vi "Shooting Stars RT Test.vi"() -> ()   [LabVIEW 2021]
uses:
  Display Utilities/Public/Controls/2D Dimensions.ctl
  Neopixel - Host/Public/Controls/RGB Gains.ctl
  Display Utilities/Public/Controls/2D Coordinates.ctl
  Pixel/Pixel.lvclass
  C:/Git/MEMOSFET/myRIO-Neopixel/Source/RT/Display Element/Display Element.lvclass
  <vilib>/numeric/Random Number (Range) U64.vi
  <vilib>/numeric/Random Number (Range) I64.vi
  <vilib>/numeric/sub_Random U32.vi
  <vilib>/FPGAPlugInAG/myRIO-1900/niLvFpga_Open_myRIO-1900.vi
  <vilib>/rvi/interface/common/dynamic/niFpgaDynamicAddResources.vi
  <vilib>/FPGAPlugInAG/Dynamic/niLvFpga_Close_Dynamic.vi
  <vilib>/rvi/interface/nirviOpenFPGA/nirviOpenFPGA.xnode
  FPGA Bitfiles/Test Neopixel.lvbitx
  <vilib>/rvi/interface/nirviCloseFPGA/nirviCloseFPGA.xnode
  Neopixel - Host/Neopixel - Host.lvclass
  Display Utilities/Display Utilities.lvlib
  Display Manager/Display Manager.lvclass
panel:
  out "Frame":u32[][](array[colorbox])
  in  "Intensity":sgl(slide)=0.5 scale=0.0..1.0
  in  "FPS":u32(slide)=40 scale=0.0..500.0
  in  "stop":bool
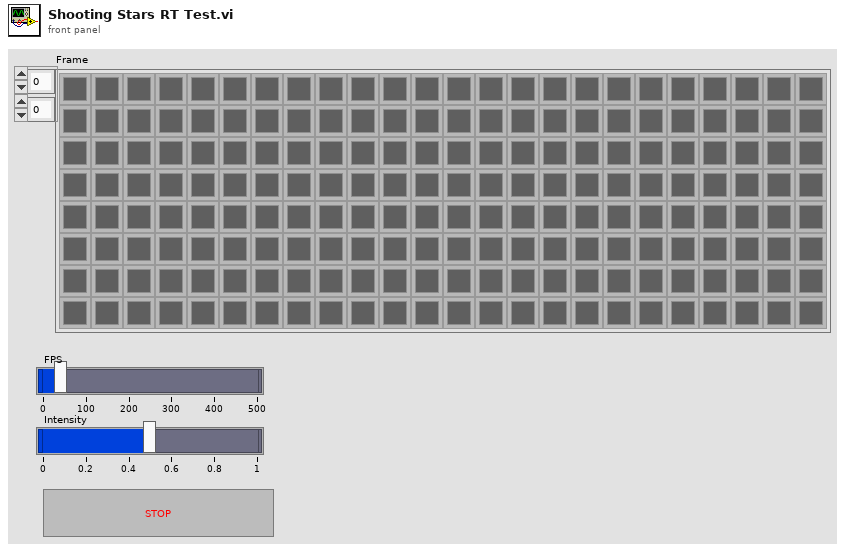
[diagram p1: front panel]
types:
  T1 = typedef "Display Utilities.lvlib/2D Dimensions.ctl" = cluster{"Width":i32, "Height":i32}
  T2 = typedef "Neopixel - Host.lvclass/RGB Gains.ctl" = cluster{"Red":sgl, "Green":sgl, "Blue":sgl}
  T3 = typedef "Display Utilities.lvlib/2D Coordinates.ctl" = cluster{"X":i32, "Y":i32}
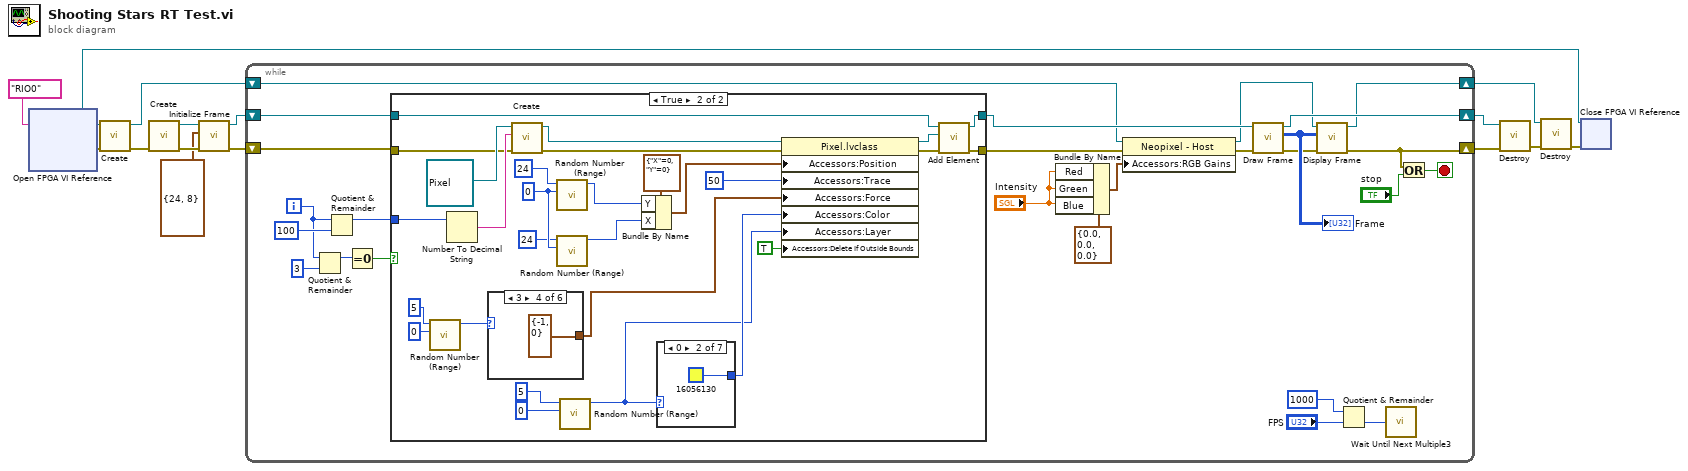
[diagram p0: block diagram]
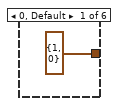
[diagram p3: hidden frame]
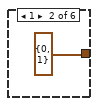
[diagram p4: hidden frame]
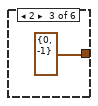
[diagram p5: hidden frame]
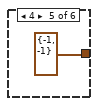
[diagram p6: hidden frame]
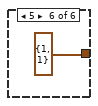
[diagram p7: hidden frame]
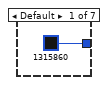
[diagram p8: hidden frame]
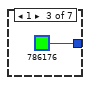
[diagram p9: hidden frame]
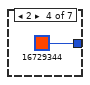
[diagram p10: hidden frame]
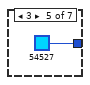
[diagram p11: hidden frame]
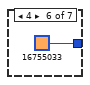
[diagram p12: hidden frame]
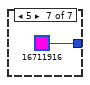
[diagram p13: hidden frame]
diagram:
  n1 = xnode "Open FPGA VI Reference"("resource name"=tag "RIO0") -> ("FPGA VI Reference Out"=w5:refnum<k20>, "error out"=w7:errorcluster)  [unwired: 1 in]
  n2 = call "Create.vi"("Error In"=w7, "FPGA Reference"=w5) -> ("Error Out"=w4:errorcluster, "Screen Out"=w3:refnum<class "Neopixel - Host.lvclass">)  [unwired: 8 in]
  n3 = call "Create.vi"("Error In"=w4) -> ("Error Out"=w14:errorcluster, "Display Manager Out"=w15:refnum<class "Display Manager.lvclass">)  [unwired: 9 in]
  n4 = call "Initialize Frame.vi"("Error In"=w14, "Size"=T1 {"Width"=24, "Height"=8}, "Display Manager In"=w15) -> ("Error Out"=w10:errorcluster, "Display Manager Out"=w9:refnum<class "Display Manager.lvclass">)  [unwired: 7 in]
  n5 = while {
    shift-right: [w32] -> w11
    shift-left: w9 -> [w41]
    shift-right: [w19] -> w12
    shift-left: w10 -> [w40]
    shift-right: [w21] -> w1
    shift-left: w3 -> [w22]
    i -> [w35]
    stop <- w31 stop-if-true
    n6 = Quotient & Remainder(x=w35, y=3) -> (x-y*floor(x/y)=w38:i32)  [unwired: 1 out]
    n7 = Quotient & Remainder(x=w35, y=100) -> (x-y*floor(x/y)=w34:i32)  [unwired: 1 out]
    n8 = Equal To 0?(x=w38) -> (x = 0?=w37:bool)
    n9 = case shown="True" w37 {
      tunnel: w40 -> [w42 w46]
      tunnel: w34 -> [_ w71]
      tunnel: w41 -> [w43 w70]
      tunnel: [w43 w69] -> w33
      tunnel: [w42 w68] -> w17
      frame False {
      }
      frame True {
        w60 = u64 0 ("lower bound (0)")
        n10 = call-poly <vilib>:"Random Number (Range).vi"("lower bound (0)"=u64 0, "upper bound (100)"=u64 5) -> ("number"=w52:u64)  [unwired: 9 in]
        n11 = Number To Decimal String(number=w71) -> (decimal integer string=w47:string)  [unwired: 1 in]
        n12 = case shown="3" w52 {
          tunnel: [T3 {"X"=1, "Y"=0} ("Position") T3 {"X"=0, "Y"=1} ("Position") T3 {"X"=0, "Y"=-1} ("Position") T3 {"X"=-1, "Y"=0} ("Position") T3 {"X"=-1, "Y"=-1} ("Position") T3 {"X"=1, "Y"=1} ("Position")] -> w51
          frame 0, Default {
          }
          frame 1 {
          }
          frame 2 {
          }
          frame 3 {
          }
          frame 4 {
          }
          frame 5 {
          }
        }
        n13 = call-dynamic "Create.vi"("Error In"=w46, "Tag"=w47, "Pixel In"=refnum<class "Pixel.lvclass"> refnum ("Pixel.lvclass")) -> ("Error Out"=w44:errorcluster, "Pixel Out"=w45:refnum<class "Pixel.lvclass">)  [unwired: 7 in]
        n14 = call-poly <vilib>:"Random Number (Range).vi"("lower bound (0)"=w60, "upper bound (100)"=u64 24) -> ("number"=w64:u64)  [unwired: 9 in]
        n15 = call-poly <vilib>:"Random Number (Range).vi"("lower bound (0)"=w60, "upper bound (100)"=u64 24) -> ("number"=w63:u64)  [unwired: 9 in]
        n16 = call-poly <vilib>:"Random Number (Range).vi"("lower bound (-100)"=i64 0, "upper bound (100)"=i64 5) -> ("number"=w56:i64)  [unwired: 9 in]
        n17 = Bundle By Name(cluster=T3 {"X"=0, "Y"=0} ("Position"), "Y"=w64, "X"=w63) -> (w62:T3)
        n18 = case shown="0" w56 {
          tunnel: [u32 1315860 ("Color") u32 16056130 ("Color") u32 786176 ("Color") u32 16729344 ("Color") u32 54527 ("Color") u32 16755033 ("Color") u32 16711916 ("Color")] -> w57
          frame Default {
          }
          frame 0 {
          }
          frame 1 {
          }
          frame 2 {
          }
          frame 3 {
          }
          frame 4 {
          }
          frame 5 {
          }
        }
        n19 = property class="Pixel.lvclass"(reference=w45, error in=w44, "Accessors:Position"=w62, "Accessors:Trace"=50 ("Trace"), "Accessors:Force"=w51, "Accessors:Color"=w57, "Accessors:Layer"=w56, "Accessors:Delete If Outside Bounds"=TRUE ("Delete If Outside Bounds")) -> (reference out=w67:refnum<class "Pixel.lvclass">, error out=w66:errorcluster)
        n20 = call "Add Element.vi"("Error In"=w66, "New Element"=w67, "Display Manager In"=w70) -> ("Error Out"=w68:errorcluster, "Display Manager Out"=w69:refnum<class "Display Manager.lvclass">)  [unwired: 7 in]
      }
    }
    n21 = Bundle By Name(cluster=T2 {"Red"=0.0, "Green"=0.0, "Blue"=0.0} ("RGB Gains"), "Red"="Intensity", "Green"="Intensity", "Blue"="Intensity") -> (w25:T2)
    n22 = property class="Neopixel - Host"(reference=w22, error in=w17, "Accessors:RGB Gains"=w25) -> (reference out=w24:refnum<class "Neopixel - Host.lvclass">, error out=w18:errorcluster)
    n23 = call "Draw Frame.vi"("Error In"=w18, "Display Manager In"=w33) -> ("Error Out"=w16:errorcluster, "Frame"=w20:u32[][], "Display Manager Out"=w32:refnum<class "Display Manager.lvclass">)  [unwired: 7 in]
    "Frame" <- w20
    n24 = call "Display Frame.vi"("Error In"=w16, "Frame"=w20, "Display In"=w24) -> ("Error Out"=w19:errorcluster, "Display Out"=w21:refnum<class "Neopixel - Host.lvclass">)  [unwired: 7 in]
    n25 = Quotient & Remainder(x=u32 1000 ("y"), y="FPS") -> (floor(x/y)=w28:u32)  [unwired: 1 out]
    n26 = call "Wait Until Next Multiple3"("Count(mSec)"=w28) -> ()  [unwired: 1 out]
    n27 = Or(x=w19, y="stop") -> (x .or. y?=w31:bool)
  }
  n28 = call "Destroy.vi"("Error In"=w12, "Display Manager In"=w11) -> ("Error Out"=w2:errorcluster)  [unwired: 9 in]
  n29 = call "Destroy.vi"("Error In"=w2, "Display In"=w1) -> ("Error Out"=w6:errorcluster)  [unwired: 9 in]
  n30 = xnode "Close FPGA VI Reference"("FPGA VI Reference In"=w5, "error in"=w6) -> ()  [unwired: 1 out]
